vi "Test Base Namer Default Behavior.vi"(11 "Test Case In":refnum<class "Namer Tests.lvclass">) -> (0 "error out":errorcluster, 3 "Test Case Out":refnum<class "Namer Tests.lvclass">)   [LabVIEW 2020, in "Namer Tests.lvclass"]
uses:
  Namer Tests.lvclass
  C:/Program Files/National Instruments/LabVIEW 2026/vi.lib/Astemes/LUnit/Test Case.lvclass
  Source/Approval Tests/Namer/Namer.lvclass
  Source/Approval Tests/Naming Data/Naming Data.lvclass
  Source/Approval Tests/Naming Data/Naming Data.lvclass/Naming Data.ctl
  <vilib>/Astemes/LUnit/Test Case.lvclass/Test Case.ctl
  4993e8ee-a06a-463a-9684-69129f64d5ce.vi
  9ab5aa2e-c9e0-474c-82b3-5a65eb4534de.vi
  Source/Approval Tests/Naming Data/Write Test VI Name.vi
  <vilib>/Astemes/LUnit/Core/LUnit Test Case/Private/Append Pass Result.vi
  <vilib>/Astemes/LUnit/Core/LUnit Test Case/Private/Append Fail Result.vi
  4993e8ee-a06a-463a-9684-69129f64d5ce.vi/9c5d11cd-9439-4240-a1ee-d9baace9c924.vi
  9ab5aa2e-c9e0-474c-82b3-5a65eb4534de.vi/9c5d11cd-9439-4240-a1ee-d9baace9c924.vi
  <vilib>/Astemes/LUnit/Core/LUnit Test Case/Private/Run In UI.vi
  <vilib>/Utility/error.llb/Clear Errors.vi
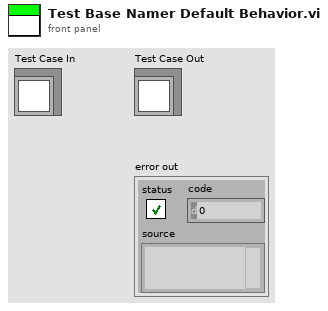
[diagram p1: front panel]
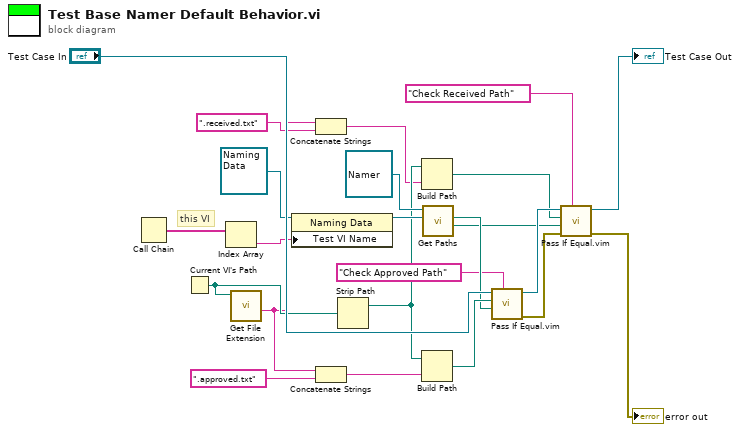
[diagram p0: block diagram]
diagram:
  # "this VI"
  n1 = Call Chain() -> (call chain=w18:string[])
  n2 = Current VI's Path() -> (path=w15:path)
  n3 = Index Array(array=w18) -> (element=w17:string)  [unwired: 1 in]
  n4 = call <vilib>:"Get File Extension.vi"("file"=w15) -> ("filename without extension"=w13:string)  [unwired: 6 in, 4 out]
  n5 = property on="Property Node" class="Naming Data"(reference=refnum<class "Naming Data.lvclass"> refnum ("Naming Data"), "Test VI Name"=w17) -> (reference out=w16:refnum<class "Naming Data.lvclass">)  [unwired: 1 in, 1 out]
  n6 = Concatenate Strings(w13, ".received.txt" ("string")) -> (w10:string)
  n7 = Concatenate Strings(w13, ".approved.txt" ("string")) -> (w9:string)
  n8 = Strip Path(path=w15) -> (stripped path=w14:path)  [unwired: 1 out]
  n9 = Build Path(base path=w14, name or relative path=w10) -> (appended path=w3:path)
  n10 = Build Path(base path=w14, name or relative path=w9) -> (appended path=w8:path)
  n11 = call-dynamic "Get Paths.vi"("Naming Data"=w16, "Namer in"=refnum<class "Namer.lvclass"> refnum ("Approval Tests:Namer")) -> ("Received Path"=w2:path, "Approved Path"=w7:path)  [unwired: 6 in, 2 out]
  n12 = call "Pass If Equal.vim"("Description"="Check Approved Path", "Actual"=w7, "Expected"=w8, "LUnit Test Case In"="Test Case In") -> ("error out"=w22:errorcluster, "LUnit Test Case Out"=w5:refnum<class "Namer Tests.lvclass">)  [unwired: 6 in]
  n13 = call "Pass If Equal.vim"("Description"="Check Received Path" ("Label (VI Title)"), "error in (no error)"=w22, "Actual"=w2, "Expected"=w3, "LUnit Test Case In"=w5) -> ("error out"=→"error out":errorcluster, "LUnit Test Case Out"=→"Test Case Out":refnum<class "Namer Tests.lvclass">)  [unwired: 5 in]
